vi "ROI entry-Rectangle to XY Point.vi"(11 "Rectangle":T1) -> (3 "XY":cluster{"X":i32, "Y":i32})   [LabVIEW 2013]
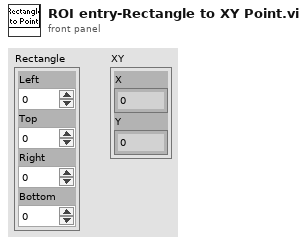
[diagram p1: front panel]
types:
  T1 = cluster{"Left":i32, "Top":i32, "Right":i32, "Bottom":i32}
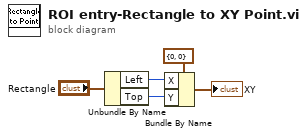
[diagram p0: block diagram]
diagram:
  n1 = Unbundle By Name("Rectangle") -> ("Left"=w3:i32, "Top"=w4:i32)
  n2 = Bundle By Name(cluster=cluster{"X":i32, "Y":i32} {"X"=0, "Y"=0} ("Point"), "X"=w3, "Y"=w4) -> (→"XY":cluster{"X":i32, "Y":i32})
